vi "AverageMarkers (SubVI).vi"(1 "Markers":T1[][](array[typedef])) -> (0 "Avg Markers":T1[](array[typedef]))   [LabVIEW 2021]
uses:
  ctrOWLMarker.ctl
  <vilib>/Analysis/baseanly.llb/Mean (DBL).vi
  <vilib>/Analysis/NI_AALBase.lvlib
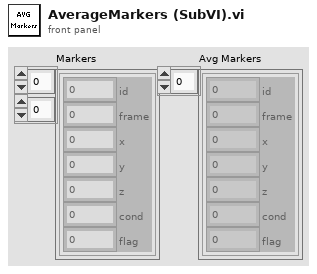
[diagram p1: front panel]
types:
  T1 = typedef "ctrOWLMarker.ctl" = cluster{"id":i32, "frame":i32, "x":sgl, "y":sgl, "z":sgl, "cond":sgl, "flag":u32}
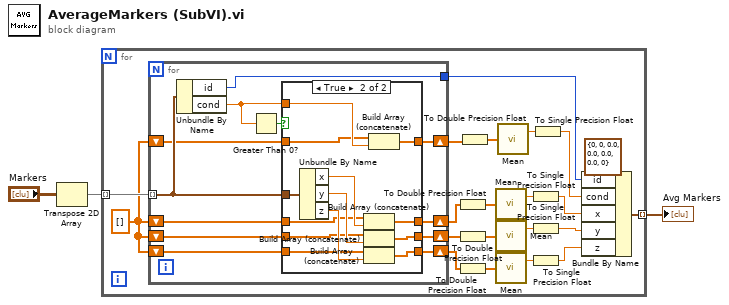
[diagram p0: block diagram]
diagram:
  n1 = Transpose 2D Array(2D array="Markers") -> (transposed array=w1:T1[][])
  n2 = for {
    tunnel: w1 -> [w24] mode=indexing
    tunnel: [w22] -> w2 mode=indexing
    w8 = sgl[] []
    n3 = for {
      tunnel: w24 -> [w35] mode=indexing
      shift-right: [w34] -> w21
      shift-left: w8 -> [w31]
      shift-right: [w33] -> w20
      shift-left: w8 -> [w30]
      shift-right: [w32] -> w19
      shift-left: w8 -> [w29]
      tunnel: [w28] -> w9
      shift-right: [w27] -> w5
      shift-left: w8 -> [w26]
      n4 = Unbundle By Name(w35) -> ("id"=w28:i32, "cond"=w25:sgl)
      n5 = Greater Than 0?(x=w25) -> (x > 0?=w36:bool)
      n6 = case shown="True" w36 {
        tunnel: w35 -> [_ w53]
        tunnel: [w40 w49] -> w34
        tunnel: [w39 w48] -> w33
        tunnel: [w38 w47] -> w32
        tunnel: w31 -> [w40 w46]
        tunnel: w30 -> [w39 w45]
        tunnel: w29 -> [w38 w44]
        tunnel: w25 -> [_ w43]
        tunnel: [w37 w42] -> w27
        tunnel: w26 -> [w37 w41]
        frame False {
        }
        frame True {
          n7 = Unbundle By Name(w53) -> ("x"=w52:sgl, "y"=w51:sgl, "z"=w50:sgl)
          n8 = Build Array (concatenate)(w46, w52) -> (w49:sgl[])
          n9 = Build Array (concatenate)(w45, w51) -> (w48:sgl[])
          n10 = Build Array (concatenate)(w44, w50) -> (w47:sgl[])
          n11 = Build Array (concatenate)(w41, w43) -> (w42:sgl[])
        }
      }
    }
    n12 = To Double Precision Float(number=w21) -> (double precision float=w18:dbl[])
    n13 = To Double Precision Float(number=w20) -> (double precision float=w17:dbl[])
    n14 = To Double Precision Float(number=w19) -> (double precision float=w16:dbl[])
    n15 = To Double Precision Float(number=w5) -> (double precision float=w6:dbl[])
    n16 = call-poly <vilib>:"Mean.vi"("X"=w18) -> ("mean"=w15:dbl)  [unwired: 1 out]
    n17 = call-poly <vilib>:"Mean.vi"("X"=w17) -> ("mean"=w14:dbl)  [unwired: 1 out]
    n18 = call-poly <vilib>:"Mean.vi"("X"=w16) -> ("mean"=w13:dbl)  [unwired: 1 out]
    n19 = call-poly <vilib>:"Mean.vi"("X"=w6) -> ("mean"=w7:dbl)  [unwired: 1 out]
    n20 = To Single Precision Float(number=w15) -> (single precision float=w12:sgl)
    n21 = To Single Precision Float(number=w14) -> (single precision float=w11:sgl)
    n22 = To Single Precision Float(number=w13) -> (single precision float=w10:sgl)
    n23 = To Single Precision Float(number=w7) -> (single precision float=w4:sgl)
    n24 = Bundle By Name(cluster=T1 {"id"=0, "frame"=0, "x"=0.0, "y"=0.0, "z"=0.0, "cond"=0.0, "flag"=0} ("OWLMarker"), "id"=w9, "cond"=w4, "x"=w12, "y"=w11, "z"=w10) -> (w22:T1)
  }
  "Avg Markers" <- w2
